vi "Store Value in TDMS File.vi"(5 "Replace name with prefix (FALSE = append)":bool, 6 "Value":variant, 7 "Prefix":string, 8 "Error In":errorcluster, 9 "channel name":string, 10 "group name":string, 11 "File Path":path) -> (0 "Error Out":errorcluster, 1 "channel name out":string, 2 "group name out":string, 3 "File Path out":path)   [LabVIEW 2021]
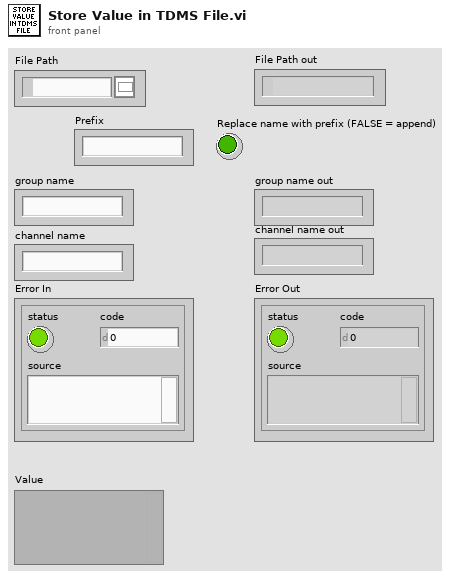
[diagram p1: front panel]
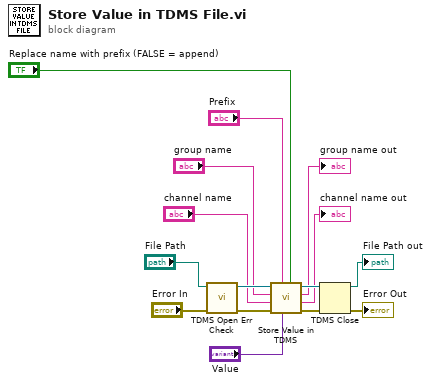
[diagram p0: block diagram]
diagram:
  n1 = call "TDMS Open Err Check.vi"("Error In"="Error In", "File Path Control"="File Path") -> ("Error Out"=w13:errorcluster, "tdms file out"=w14:refnum<k34>)  [unwired: 7 in, 1 out]
  n2 = call "Store Value in TDMS.vi"("Replace name with prefix (FALSE = append)"="Replace name with prefix (FALSE = append)", "Value"="Value", "Prefix"="Prefix", "Error In"=w13, "channel name"="channel name", "group name"="group name", "tdms file"=w14) -> ("Error Out"=w12:errorcluster, "channel name out"=→"channel name out":string, "group name out"=→"group name out":string, "tdms file out"=w11:refnum<k34>)  [unwired: 1 in]
  n3 = TDMS Close(8:w12, 11:w11) -> (0:→"Error Out":errorcluster, 3:→"File Path out":path)
